vi "Replace Named Format Specifier.vi"(8 "error in (no error)":errorcluster, 10 "data":variant, 11 "format string":string) -> (0 "error out":errorcluster, 3 "resulting string":string)   [LabVIEW 2024, in "Logging.lvlib" / "Format String.lvclass"]
uses:
  Format String.lvclass
  <vilib>/regexp/Match Regular Expression.xnode
  <vilib>/ErrorRing/Error Ring.xnode
  <userlib>/_OpenG.lib/lvdata/lvdata.llb/openg_variant.lvlib
  <vilib>/Utility/Data Type/NI_Data Type.lvlib
panel:
  # "Connector Pane"
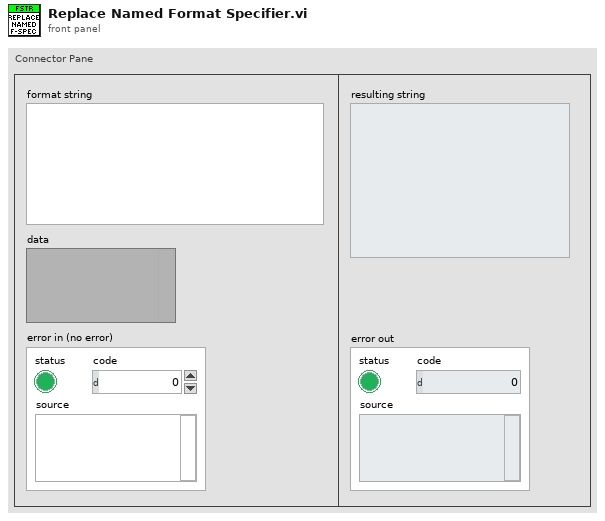
[diagram p1: front panel]
types:
  T1 = typedef "NI_Data Type.lvlib/Data Type.ctl" = enum8{"Invalid Type", "Void", "I8", "I16", "I32", "I64", "U8", "U16", "U32", "U64", "Single Float", "Double Float", "Extended Float", "Single Complex", "Double Complex", "Extended Complex", "Enum U8", "Enum U16", "Enum U32", "Enum U64", "Single Float With Unit", "Double Float With Unit", "Extended Float With Unit", "Single Complex with Unit", "Double Complex with Unit", "Extended Complex with Unit", "Boolean", "String", "Path", "Picture", "Tag", "Array", "Cluster", "Variant", "LV Variant", "Waveform", "Timestamp", "Digital Waveform", "Digital Data", "ExpressData", "Refnum", "External Data", "VI", "Poly VI", "LabVIEW Class Instance", "Fixed Point", "Set Collection", "Map Collection"}
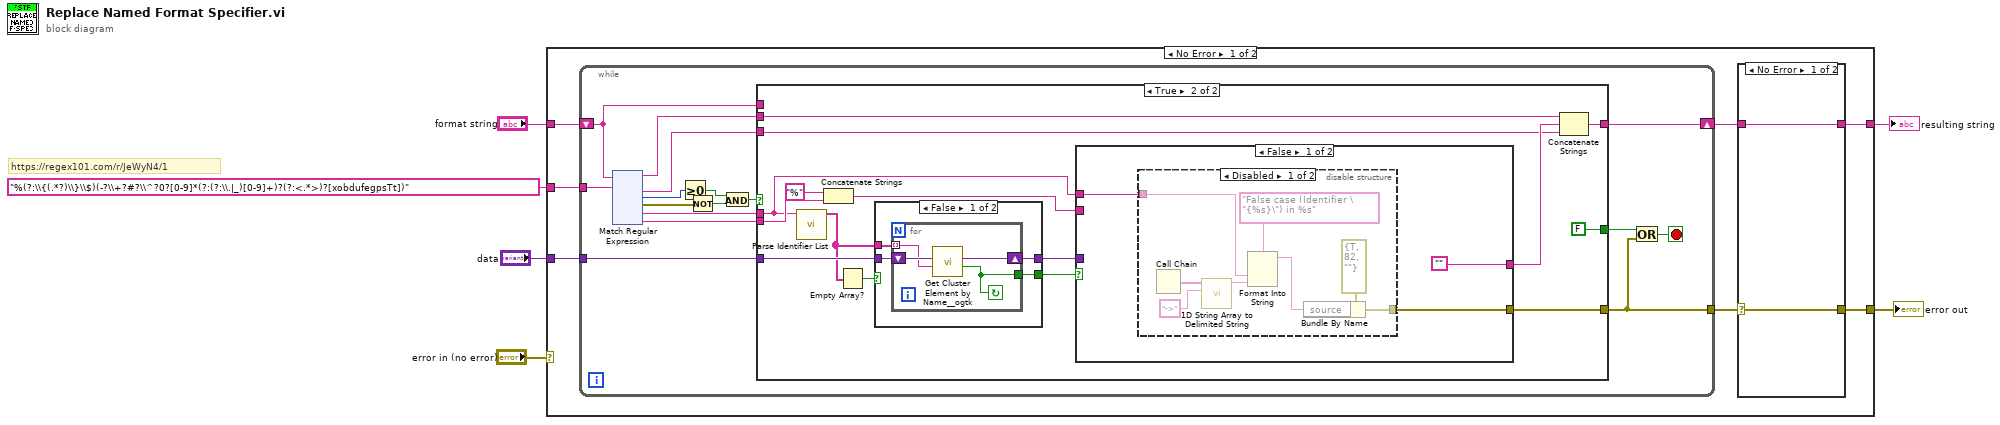
[diagram p0: block diagram]
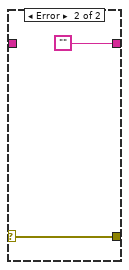
[diagram p2: hidden frame]
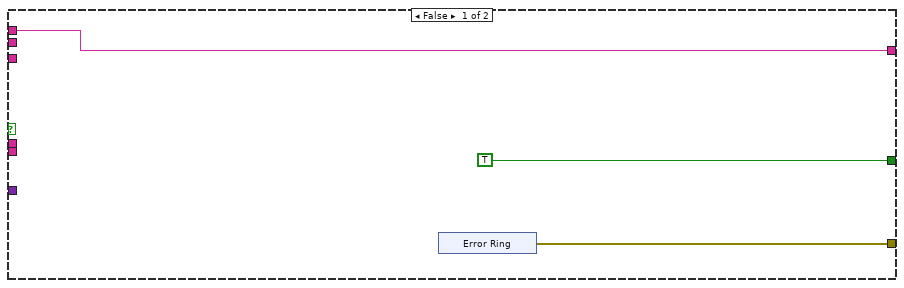
[diagram p3: hidden frame]
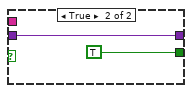
[diagram p4: hidden frame]
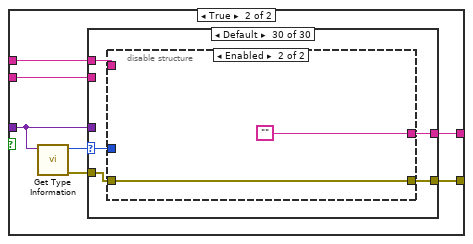
[diagram p6: hidden frame]
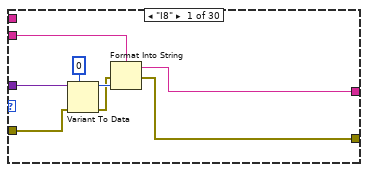
[diagram p7: hidden frame]
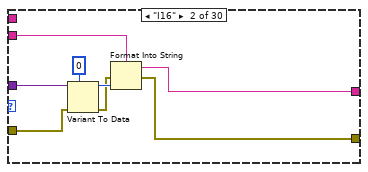
[diagram p8: hidden frame]
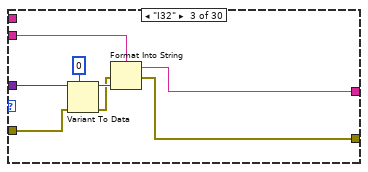
[diagram p9: hidden frame]
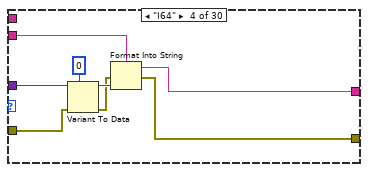
[diagram p10: hidden frame]
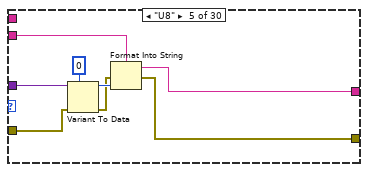
[diagram p11: hidden frame]
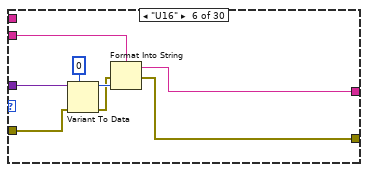
[diagram p12: hidden frame]
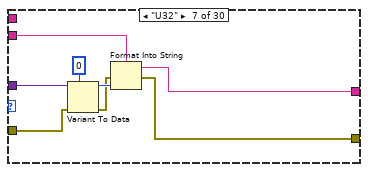
[diagram p13: hidden frame]
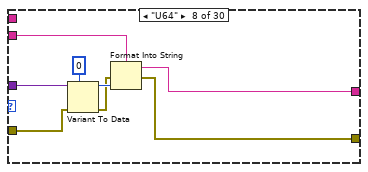
[diagram p14: hidden frame]
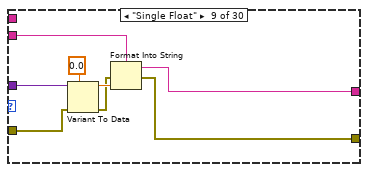
[diagram p15: hidden frame]
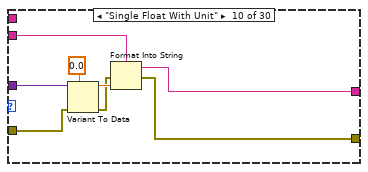
[diagram p16: hidden frame]
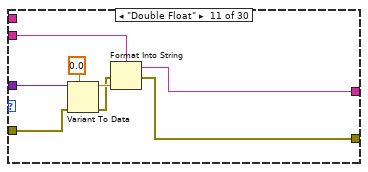
[diagram p17: hidden frame]
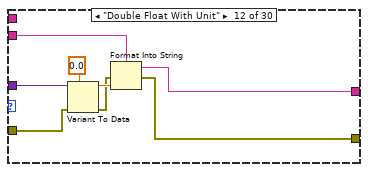
[diagram p18: hidden frame]
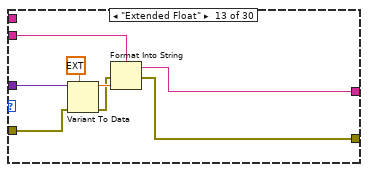
[diagram p19: hidden frame]
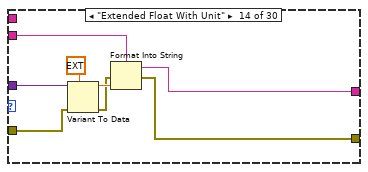
[diagram p20: hidden frame]
diagram:
  # "https://regex101.com/r/JeWyN4/1"
  n1 = case shown="No Error" "error in (no error)" {
    selector: "error in (no error)" -> [_ w488]
    tunnel: "format string" -> [w13 _]
    tunnel: "%(?:\\{(.*?)\\}\\$)(-?\\+?#?\\^?0?[0-9]*(?:(?:\\.|_)[0-9]+)?(?:<.*>)?[xobdufegpsTt])" -> [w12 _]
    tunnel: "data" -> [w11 _]
    tunnel: [w9 w488] -> w3
    tunnel: [w8 ""] -> w2
    frame No Error {
      n2 = while {
        tunnel: w12 -> [w32]
        tunnel: w11 -> [w30]
        shift-right: [w27] -> w7
        shift-left: w13 -> [w18]
        tunnel: [w19] -> w10
        stop <- w20 stop-if-true
        n3 = xnode "Match Regular Expression"("input string"=w18, "regular expression"=w32) -> ("before match"=w29:string, "after match"=w28:string, "offset past match"=w26:i32, "error out"=w25:errorcluster, "submatch 1"=w33:string, "submatch 2"=w31:string)  [unwired: 4 in, 1 out]
        n4 = Greater Or Equal To 0?(x=w26) -> (x >= 0?=w24:bool)
        n5 = Not(x=w25) -> (.not. x?=w23:bool)
        n6 = And(x=w24, y=w23) -> (x .and. y?=w22:bool)
        n7 = case shown="True" w22 {
          tunnel: w33 -> [_ w160]
          tunnel: w31 -> [_ w171]
          tunnel: w30 -> [_ w161]
          tunnel: w29 -> [_ w167]
          tunnel: w28 -> [_ w165]
          tunnel: [w156 w164] -> w27
          tunnel: [TRUE FALSE] -> w21
          tunnel: [w154 w162] -> w19
          tunnel: w18 -> [w156 _]
          frame False {
            n8 = xnode "Error Ring"() -> ("error out"=w154:errorcluster)
          }
          frame True {
            n9 = call "Parse Identifier List.vi"("string"=w160) -> ("identifier list"=w159:string[])  [unwired: 10 in]
            n10 = Concatenate Strings("%" ("string"), w171) -> (w168:string)
            n11 = Empty Array?(array=w159) -> (empty?=w158:bool)
            n12 = case shown="False" w158 {
              tunnel: w159 -> [w176 _]
              tunnel: [w175 TRUE ("found?")] -> w170
              tunnel: [w174 w182] -> w169
              tunnel: w161 -> [w173 w182]
              frame False {
                n13 = for {
                  tunnel: w176 -> [w179] mode=indexing
                  shift-right: [w178] -> w174
                  shift-left: w173 -> [w180]
                  tunnel: [w177] -> w175
                  stop <- w177 continue-if-true
                  n14 = call <userlib>:"Get Cluster Element by Name__ogtk.vi"("Element Name"=w179, "Cluster"=w180) -> ("found?"=w177:bool, "VElement"=w178:variant)  [unwired: 7 in, 1 out]
                }
              }
              frame True {
              }
            }
            n15 = case shown="False" w170 {
              tunnel: w169 -> [_ w198]
              tunnel: ["" w199] -> w166
              tunnel: w168 -> [_ w197]
              tunnel: [w184 w196] -> w162
              tunnel: w160 -> [w183 w195]
              frame False {
                n16 = disable-structure shown="Disabled" {
                  disable-tunnel: [w187 _] -> w184
                  disable-tunnel: w183 -> [w186 _]
                  frame Disabled {
                    n17 = Call Chain() -> (call chain=w191:string[])
                    n18 = call <vilib>:"1D String Array to Delimited String.vi"("delimiter"="->", "string array"=w191) -> ("delimited string"=w192:string)  [unwired: 9 in]
                    n19 = Format Into String(format string="False case (Identifier \"{%s}\") in %s", w186, w192) -> (resulting string=w188:string)  [unwired: 2 in, 1 out]
                    n20 = Bundle By Name(cluster=errorcluster {"status"=TRUE, "code"=82, "source"=""} ("error constant"), "source"=w188) -> (w187:errorcluster)
                  }
                  frame Enabled {
                  }
                }
              }
              frame True {
                n21 = call <vilib>:"Get Type Information.vi"("variant"=w198) -> ("error out"=w194:errorcluster, "type"=w200:T1)  [unwired: 6 in, 3 out]
                n22 = case shown="Default" w200 {
                  selector: w200 -> [_ _ _ _ _ _ _ _ _ _ _ _ _ _ _ _ _ _ _ _ _ _ _ _ _ _ _ _ _ w472]
                  tunnel: [w203 w211 w219 w227 w235 w243 w251 w259 w267 w275 w283 w291 w299 w307 w315 w323 w331 w339 w347 w355 w364 w383 w402 w421 w439 w447 w455 w463 "" w475] -> w199
                  tunnel: w198 -> [w208 w216 w224 w232 w240 w248 w256 w264 w272 w280 w288 w296 w304 w312 w320 w328 w336 w344 w352 w360 w367 w386 w405 w424 w444 w452 w460 w468 _ _]
                  tunnel: w197 -> [w206 w214 w222 w230 w238 w246 w254 w262 w270 w278 w286 w294 w302 w310 w318 w326 w334 w342 w350 w358 w366 w385 w404 w423 w442 w450 w458 w466 _ _]
                  tunnel: [w204 w212 w220 w228 w236 w244 w252 w260 w268 w276 w284 w292 w300 w308 w316 w324 w332 w340 w348 w356 w362 w381 w400 w419 w440 w448 w456 w464 w469 w474] -> w196
                  tunnel: w195 -> [_ _ _ _ _ _ _ _ _ _ _ _ _ _ _ _ _ _ _ _ _ _ _ _ _ _ _ _ _ w473]
                  tunnel: w194 -> [w201 w209 w217 w225 w233 w241 w249 w257 w265 w273 w281 w289 w297 w305 w313 w321 w329 w337 w345 w353 w361 w380 w399 w418 w437 w445 w453 w461 w469 w471]
                  frame "I8" {
                    n23 = Variant To Data(error in=w201, type=i8 0, Variant=w208) -> (data=w205:i8, error out=w202:errorcluster)
                    n24 = Format Into String(format string=w206, error in=w202, w205) -> (resulting string=w203:string, error out=w204:errorcluster)  [unwired: 1 in]
                  }
                  frame "I16" {
                    n25 = Variant To Data(error in=w209, type=i16 0, Variant=w216) -> (data=w213:i16, error out=w210:errorcluster)
                    n26 = Format Into String(format string=w214, error in=w210, w213) -> (resulting string=w211:string, error out=w212:errorcluster)  [unwired: 1 in]
                  }
                  frame "I32" {
                    n27 = Variant To Data(error in=w217, type=0, Variant=w224) -> (data=w221:i32, error out=w218:errorcluster)
                    n28 = Format Into String(format string=w222, error in=w218, w221) -> (resulting string=w219:string, error out=w220:errorcluster)  [unwired: 1 in]
                  }
                  frame "I64" {
                    n29 = Variant To Data(error in=w225, type=i64 0, Variant=w232) -> (data=w229:i64, error out=w226:errorcluster)
                    n30 = Format Into String(format string=w230, error in=w226, w229) -> (resulting string=w227:string, error out=w228:errorcluster)  [unwired: 1 in]
                  }
                  frame "U8" {
                    n31 = Variant To Data(error in=w233, type=u8 0, Variant=w240) -> (data=w237:u8, error out=w234:errorcluster)
                    n32 = Format Into String(format string=w238, error in=w234, w237) -> (resulting string=w235:string, error out=w236:errorcluster)  [unwired: 1 in]
                  }
                  frame "U16" {
                    n33 = Variant To Data(error in=w241, type=u16 0, Variant=w248) -> (data=w245:u16, error out=w242:errorcluster)
                    n34 = Format Into String(format string=w246, error in=w242, w245) -> (resulting string=w243:string, error out=w244:errorcluster)  [unwired: 1 in]
                  }
                  frame "U32" {
                    n35 = Variant To Data(error in=w249, type=u32 0, Variant=w256) -> (data=w253:u32, error out=w250:errorcluster)
                    n36 = Format Into String(format string=w254, error in=w250, w253) -> (resulting string=w251:string, error out=w252:errorcluster)  [unwired: 1 in]
                  }
                  frame "U64" {
                    n37 = Variant To Data(error in=w257, type=u64 0, Variant=w264) -> (data=w261:u64, error out=w258:errorcluster)
                    n38 = Format Into String(format string=w262, error in=w258, w261) -> (resulting string=w259:string, error out=w260:errorcluster)  [unwired: 1 in]
                  }
                  frame "Single Float" {
                    n39 = Variant To Data(error in=w265, type=sgl 0.0, Variant=w272) -> (data=w269:sgl, error out=w266:errorcluster)
                    n40 = Format Into String(format string=w270, error in=w266, w269) -> (resulting string=w267:string, error out=w268:errorcluster)  [unwired: 1 in]
                  }
                  frame "Single Float With Unit" {
                    n41 = Variant To Data(error in=w273, type=sgl 0.0, Variant=w280) -> (data=w277:sgl, error out=w274:errorcluster)
                    n42 = Format Into String(format string=w278, error in=w274, w277) -> (resulting string=w275:string, error out=w276:errorcluster)  [unwired: 1 in]
                  }
                  frame "Double Float" {
                    n43 = Variant To Data(error in=w281, type=0.0, Variant=w288) -> (data=w285:dbl, error out=w282:errorcluster)
                    n44 = Format Into String(format string=w286, error in=w282, w285) -> (resulting string=w283:string, error out=w284:errorcluster)  [unwired: 1 in]
                  }
                  frame "Double Float With Unit" {
                    n45 = Variant To Data(error in=w289, type=0.0, Variant=w296) -> (data=w293:dbl, error out=w290:errorcluster)
                    n46 = Format Into String(format string=w294, error in=w290, w293) -> (resulting string=w291:string, error out=w292:errorcluster)  [unwired: 1 in]
                  }
                  frame "Extended Float" {
                    n47 = Variant To Data(error in=w297, type=ext 0.0, Variant=w304) -> (data=w301:ext, error out=w298:errorcluster)
                    n48 = Format Into String(format string=w302, error in=w298, w301) -> (resulting string=w299:string, error out=w300:errorcluster)  [unwired: 1 in]
                  }
                  frame "Extended Float With Unit" {
                    n49 = Variant To Data(error in=w305, type=ext 0.0, Variant=w312) -> (data=w309:ext, error out=w306:errorcluster)
                    n50 = Format Into String(format string=w310, error in=w306, w309) -> (resulting string=w307:string, error out=w308:errorcluster)  [unwired: 1 in]
                  }
                  frame "Single Complex" {
                    n51 = Variant To Data(error in=w313, type=csg 0.0+0.0i, Variant=w320) -> (data=w317:csg, error out=w314:errorcluster)
                    n52 = Format Into String(format string=w318, error in=w314, w317) -> (resulting string=w315:string, error out=w316:errorcluster)  [unwired: 1 in]
                  }
                  frame "Single Complex with Unit" {
                    n53 = Variant To Data(error in=w321, type=csg 0.0+0.0i, Variant=w328) -> (data=w325:csg, error out=w322:errorcluster)
                    n54 = Format Into String(format string=w326, error in=w322, w325) -> (resulting string=w323:string, error out=w324:errorcluster)  [unwired: 1 in]
                  }
                  frame "Double Complex" {
                    n55 = Variant To Data(error in=w329, type=cdb 0.0+0.0i, Variant=w336) -> (data=w333:cdb, error out=w330:errorcluster)
                    n56 = Format Into String(format string=w334, error in=w330, w333) -> (resulting string=w331:string, error out=w332:errorcluster)  [unwired: 1 in]
                  }
                  frame "Double Complex with Unit" {
                    n57 = Variant To Data(error in=w337, type=cdb 0.0+0.0i, Variant=w344) -> (data=w341:cdb, error out=w338:errorcluster)
                    n58 = Format Into String(format string=w342, error in=w338, w341) -> (resulting string=w339:string, error out=w340:errorcluster)  [unwired: 1 in]
                  }
                  frame "Extended Complex" {
                    n59 = Variant To Data(error in=w345, type=cxt 0.0+0.0i, Variant=w352) -> (data=w349:cxt, error out=w346:errorcluster)
                    n60 = Format Into String(format string=w350, error in=w346, w349) -> (resulting string=w347:string, error out=w348:errorcluster)  [unwired: 1 in]
                  }
                  frame "Extended Complex with Unit" {
                    n61 = Variant To Data(error in=w353, type=cxt 0.0+0.0i, Variant=w360) -> (data=w357:cxt, error out=w354:errorcluster)
                    n62 = Format Into String(format string=w358, error in=w354, w357) -> (resulting string=w355:string, error out=w356:errorcluster)  [unwired: 1 in]
                  }
                  frame "Enum U8" {
                    n63 = call <userlib>:"Get Strings from Enum__ogtk.vi"("error in (no error)"=w361, "Enum"=w367) -> ("error out"=w369:errorcluster, "String Value"=w368:string)  [unwired: 6 in, 2 out]
                    n64 = Format Into String(format string=w366, error in=w369, w368) -> (resulting string=w363:string, error out=w365:errorcluster)  [unwired: 1 in]
                    n65 = case shown="Error .." w365 {
                      selector: w365 -> [w370 _]
                      tunnel: w367 -> [_ w379]
                      tunnel: w366 -> [_ w375]
                      tunnel: [w371 w374] -> w364
                      tunnel: w363 -> [w371 _]
                      tunnel: [w370 w373] -> w362
                      tunnel: w361 -> [_ w372]
                      frame No Error {
                      }
                      frame Error {
                        n66 = Variant To Data(error in=w372, type=u8 0, Variant=w379) -> (data=w378:u8, error out=w376:errorcluster)
                        n67 = Format Into String(format string=w375, error in=w376, w378) -> (resulting string=w374:string, error out=w373:errorcluster)  [unwired: 1 in]
                      }
                    }
                  }
                  frame "Enum U16" {
                    n68 = call <userlib>:"Get Strings from Enum__ogtk.vi"("error in (no error)"=w380, "Enum"=w386) -> ("error out"=w388:errorcluster, "String Value"=w387:string)  [unwired: 6 in, 2 out]
                    n69 = Format Into String(format string=w385, error in=w388, w387) -> (resulting string=w382:string, error out=w384:errorcluster)  [unwired: 1 in]
                    n70 = case shown="Error .." w384 {
                      selector: w384 -> [w389 _]
                      tunnel: w386 -> [_ w398]
                      tunnel: w385 -> [_ w394]
                      tunnel: [w390 w393] -> w383
                      tunnel: w382 -> [w390 _]
                      tunnel: [w389 w392] -> w381
                      tunnel: w380 -> [_ w391]
                      frame No Error {
                      }
                      frame Error {
                        n71 = Variant To Data(error in=w391, type=u16 0, Variant=w398) -> (data=w397:u16, error out=w395:errorcluster)
                        n72 = Format Into String(format string=w394, error in=w395, w397) -> (resulting string=w393:string, error out=w392:errorcluster)  [unwired: 1 in]
                      }
                    }
                  }
                  frame "Enum U32" {
                    n73 = call <userlib>:"Get Strings from Enum__ogtk.vi"("error in (no error)"=w399, "Enum"=w405) -> ("error out"=w407:errorcluster, "String Value"=w406:string)  [unwired: 6 in, 2 out]
                    n74 = Format Into String(format string=w404, error in=w407, w406) -> (resulting string=w401:string, error out=w403:errorcluster)  [unwired: 1 in]
                    n75 = case shown="Error .." w403 {
                      selector: w403 -> [w408 _]
                      tunnel: w405 -> [_ w417]
                      tunnel: w404 -> [_ w413]
                      tunnel: [w409 w412] -> w402
                      tunnel: w401 -> [w409 _]
                      tunnel: [w408 w411] -> w400
                      tunnel: w399 -> [_ w410]
                      frame No Error {
                      }
                      frame Error {
                        n76 = Variant To Data(error in=w410, type=u32 0, Variant=w417) -> (data=w416:u32, error out=w414:errorcluster)
                        n77 = Format Into String(format string=w413, error in=w414, w416) -> (resulting string=w412:string, error out=w411:errorcluster)  [unwired: 1 in]
                      }
                    }
                  }
                  frame "Enum U64" {
                    n78 = call <userlib>:"Get Strings from Enum__ogtk.vi"("error in (no error)"=w418, "Enum"=w424) -> ("error out"=w426:errorcluster, "String Value"=w425:string)  [unwired: 6 in, 2 out]
                    n79 = Format Into String(format string=w423, error in=w426, w425) -> (resulting string=w420:string, error out=w422:errorcluster)  [unwired: 1 in]
                    n80 = case shown="Error .." w422 {
                      selector: w422 -> [w427 _]
                      tunnel: w424 -> [_ w436]
                      tunnel: w423 -> [_ w432]
                      tunnel: [w428 w431] -> w421
                      tunnel: w420 -> [w428 _]
                      tunnel: [w427 w430] -> w419
                      tunnel: w418 -> [_ w429]
                      frame No Error {
                      }
                      frame Error {
                        n81 = Variant To Data(error in=w429, type=u64 0, Variant=w436) -> (data=w435:u64, error out=w433:errorcluster)
                        n82 = Format Into String(format string=w432, error in=w433, w435) -> (resulting string=w431:string, error out=w430:errorcluster)  [unwired: 1 in]
                      }
                    }
                  }
                  frame "Boolean" {
                    n83 = Variant To Data(error in=w437, type=FALSE, Variant=w444) -> (data=w441:bool, error out=w438:errorcluster)
                    n84 = Format Into String(format string=w442, error in=w438, w441) -> (resulting string=w439:string, error out=w440:errorcluster)  [unwired: 1 in]
                  }
                  frame "String" {
                    n85 = Variant To Data(error in=w445, type="", Variant=w452) -> (data=w449:string, error out=w446:errorcluster)
                    n86 = Format Into String(format string=w450, error in=w446, w449) -> (resulting string=w447:string, error out=w448:errorcluster)  [unwired: 1 in]
                  }
                  frame "Path" {
                    n87 = Variant To Data(error in=w453, type=path "", Variant=w460) -> (data=w457:path, error out=w454:errorcluster)
                    n88 = Format Into String(format string=w458, error in=w454, w457) -> (resulting string=w455:string, error out=w456:errorcluster)  [unwired: 1 in]
                  }
                  frame "Timestamp" {
                    n89 = Variant To Data(error in=w461, type=timestamp(0 s since 1904-01-01), Variant=w468) -> (data=w465:timestamp, error out=w462:errorcluster)
                    n90 = Format Into String(format string=w466, error in=w462, w465) -> (resulting string=w463:string, error out=w464:errorcluster)  [unwired: 1 in]
                  }
                  frame "Void" {
                  }
                  frame Default {
                    n91 = disable-structure shown="Enabled" {
                      disable-tunnel: ["" ""] -> w475
                      disable-tunnel: [w483 w486] -> w474
                      disable-tunnel: w473 -> [w478 _]
                      disable-tunnel: w472 -> [w477 _]
                      disable-tunnel: w471 -> [_ w486]
                      frame Disabled {
                        n92 = Call Chain() -> (call chain=w481:string[])
                        n93 = call <vilib>:"1D String Array to Delimited String.vi"("delimiter"="->", "string array"=w481) -> ("delimited string"=w482:string)  [unwired: 9 in]
                        n94 = Format Into String(format string="Default case (Identifier \"{%s}\" had type \"%s\") in %s", w478, w477, w482) -> (resulting string=w476:string)  [unwired: 2 in, 1 out]
                        n95 = Bundle By Name(cluster=errorcluster {"status"=TRUE, "code"=81, "source"=""} ("error constant"), "source"=w476) -> (w483:errorcluster)
                      }
                      frame Enabled {
                      }
                    }
                  }
                }
              }
            }
            n96 = Concatenate Strings(w167, w166, w165) -> (w164:string)
          }
        }
        n97 = Or(x=w21, y=w19) -> (x .or. y?=w20:bool)
      }
      n98 = case shown="No Error" w10 {
        selector: w10 -> [w15 w17]
        tunnel: [w15 w17] -> w9
        tunnel: [w14 ""] -> w8
        tunnel: w7 -> [w14 _]
        frame No Error {
        }
        frame Error {
        }
      }
    }
    frame Error {
    }
  }
  "resulting string" <- w2
  "error out" <- w3
